vi "build.vi"(0 "FixedFrameBuilder in":refnum<class "FixedFrameBuilder.lvclass">, 1 "WaitForTrigger":bool, 2 "Latency":u32, 3 "WaitForRxTimeout":u32, 4 "TriggerIRQ":bool, 5 "error in (no error)":errorcluster, 7 "Timestamp":bool) -> (14 "FixedFrameBuilder out":refnum<class "FixedFrameBuilder.lvclass">, 15 "TxFrame":T1 {"Data" format="%02x"}, 19 "error out":errorcluster)   [LabVIEW 2016, in "RTModbus.lvlib" / "FixedFrameBuilder.lvclass"]
uses:
  FixedFrameBuilder.lvclass
  DataTypes/TxFrame.ctl
  FixedFrameBuilder.lvclass/FixedFrameBuilder.ctl
  RTModbus.lvlib
  Common_RT_Utilities/U8ArrayBuilderManualIndexing/U8ArrayBuilderManualIndexing.lvclass
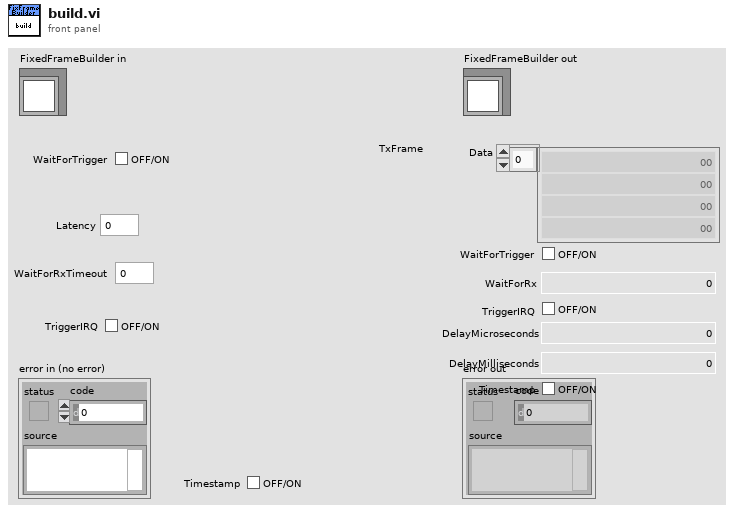
[diagram p1: front panel]
types:
  T1 = typedef "RTModbus.lvlib/TxFrame.ctl" = cluster{"Data":u8[], "WaitForTrigger":bool, "WaitForRx":u32, "TriggerIRQ":bool, "DelayMicroseconds":u16, "DelayMilliseconds":u16, "Timestamp":bool}
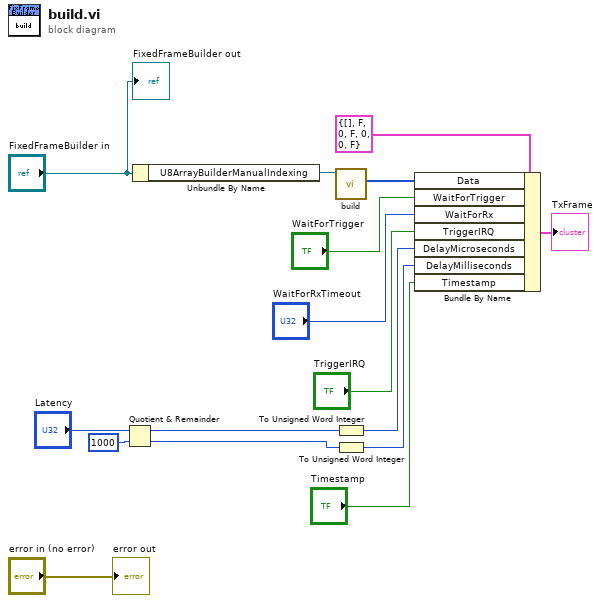
[diagram p0: block diagram]
diagram:
  n1 = Quotient & Remainder(x="Latency", y=u32 1000) -> (x-y*floor(x/y)=w10:u32, floor(x/y)=w9:u32)
  n2 = Unbundle By Name("FixedFrameBuilder in") -> ("U8ArrayBuilderManualIndexing"=w2:refnum<class "U8ArrayBuilderManualIndexing.lvclass">)
  n3 = call "build.vi"("U8ArrayBuilderManualIndexing in"=w2) -> ("Array"=w1:u8[])  [unwired: 8 in, 2 out]
  n4 = To Unsigned Word Integer(number=w10) -> (unsigned 16bit integer=w6:u16)
  n5 = To Unsigned Word Integer(number=w9) -> (unsigned 16bit integer=w5:u16)
  n6 = Bundle By Name(cluster=T1 {"Data"=[], "WaitForTrigger"=FALSE, "WaitForRx"=0, "TriggerIRQ"=FALSE, "DelayMicroseconds"=0, "DelayMilliseconds"=0, "Timestamp"=FALSE} ("Frame"), "Data"=w1, "WaitForTrigger"="WaitForTrigger", "WaitForRx"="WaitForRxTimeout", "TriggerIRQ"="TriggerIRQ", "DelayMicroseconds"=w6, "DelayMilliseconds"=w5, "Timestamp"="Timestamp") -> (→"TxFrame":T1)
  "error out" <- "error in (no error)"
  "FixedFrameBuilder out" <- "FixedFrameBuilder in"
